vi "Identify.vi"(8 "error in (no error)":errorcluster, 10 "Write IDN":bool, 11 "VISA Refnum in":refnum<visa-resource-name>) -> (0 "error out":errorcluster, 3 "VISA Refnum out":refnum<visa-resource-name>)   [LabVIEW 2011, in "Magna PSU.lvlib"]
uses:
  Magna PSU.lvlib
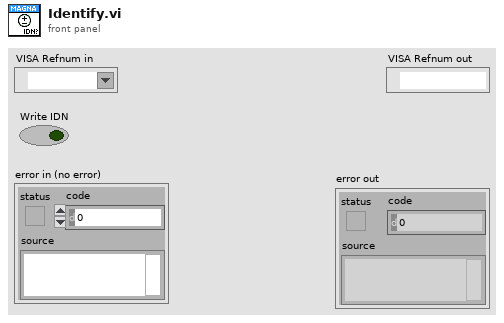
[diagram p1: front panel]
types:
  T1 = cluster{"Status":bool, "Code":i32, "Source (VI Name)":string}
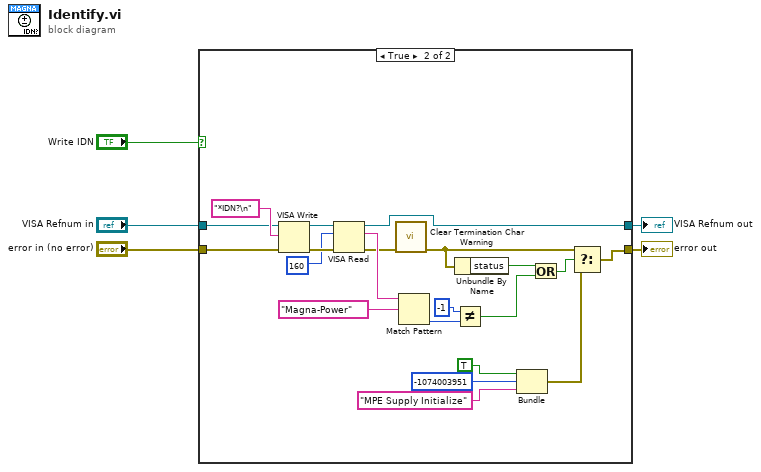
[diagram p0: block diagram]
diagram:
  n1 = case shown="True" "Write IDN" {
    tunnel: [w6 w21] -> w1
    tunnel: [w7 w8] -> w5
    tunnel: "VISA Refnum in" -> [w7 w14]
    tunnel: "error in (no error)" -> [w6 w13]
    frame False {
    }
    frame True {
      n2 = VISA Write(VISA resource name=w14, write buffer="*IDN?\n", error in (no error)=w13) -> (VISA resource name out=w24:refnum<visa-resource-name>, error out=w26:errorcluster)  [unwired: 1 out]
      n3 = VISA Read(VISA resource name=w24, byte count=u32 160, error in (no error)=w26) -> (VISA resource name out=w8:refnum<visa-resource-name>, read buffer=w11:string, error out=w10:errorcluster)  [unwired: 1 out]
      n4 = call "Clear Termination Char Warning.vi"("error in (no error)"=w10) -> ("error out"=w9:errorcluster)  [unwired: 10 in]
      n5 = Match Pattern(string=w11, regular expression="Magna-Power") -> (offset past match=w19:i32)  [unwired: 1 in, 3 out]
      n6 = Unbundle By Name(w9) -> ("status"=w22:bool)
      n7 = Not Equal?(x=-1, y=w19) -> (x != y?=w15:bool)
      n8 = Bundle("Status"=TRUE, "Code"=-1074003951, "Source (VI Name)"="MPE Supply Initialize") -> (w16:T1)  [unwired: 1 in]
      n9 = Or(x=w22, y=w15) -> (x .or. y?=w23:bool)
      n10 = Select(t=w9, s=w23, f=w16) -> (s? t:f=w21:T1)
    }
  }
  "VISA Refnum out" <- w5
  "error out" <- w1
